vi "Get Cached Result.vi"(7 "Cache string":string, 8 "error in (no error)":errorcluster, 11 "Composite Object in":refnum<class "CConfig Object.lvclass">) -> (0 "error out":errorcluster, 2 "Cached?":bool, 3 "Composite Object out":refnum<class "CConfig Object.lvclass">, 4 "Cached results":i32[](array[numeric]))   [LabVIEW 2013, in "CConfig Object.lvclass"]
doc: "Copyright 2018, Carya Automatisering, Wiebe Walstra."
uses:
  CConfig Object.lvclass
  CConfig Object.lvclass/CConfig Object.ctl
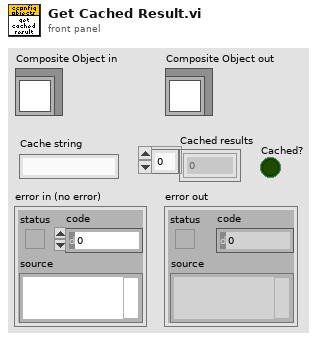
[diagram p1: front panel]
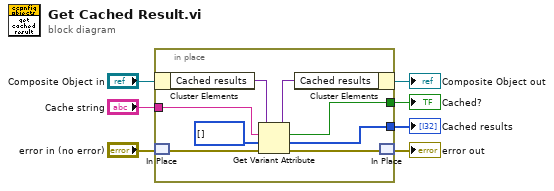
[diagram p0: block diagram]
diagram:
  n1 = in-place {
    in-place-border: [w12] -> w5
    in-place-border: [w11] -> w4
    in-place-border: "Cache string" -> [w10]
    n2 = in-place-cluster #1("Composite Object in") -> ("Cached results"=w15:variant)
    n3 = in-place-match #2("error in (no error)") -> (w9:errorcluster)
    n4 = Get Variant Attribute(Variant=w15, name=w10, default value (empty Variant)=i32[] [] ("Cached results"), error in=w9) -> (duplicate Variant=w14:variant, found=w11:bool, value=w12:i32[], error out=w8:errorcluster)
    n5 = in-place-cluster #1("Cached results"=w14) -> (→"Composite Object out":refnum<class "CConfig Object.lvclass">)
    n6 = in-place-match #2(w8) -> (→"error out":errorcluster)
  }
  "Cached?" <- w4
  "Cached results" <- w5
